vi "10.multi-dim-array.vi"() -> ()   [LabVIEW 2016]
panel:
  out "Array 3":dbl[][](array[numeric])
  out "Array 2":dbl[][](array[numeric])
  in  "Array1":dbl[][](array[numeric])
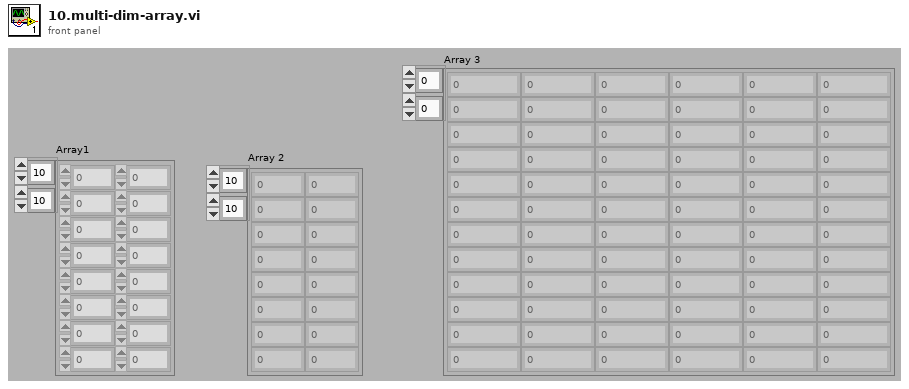
[diagram p1: front panel]
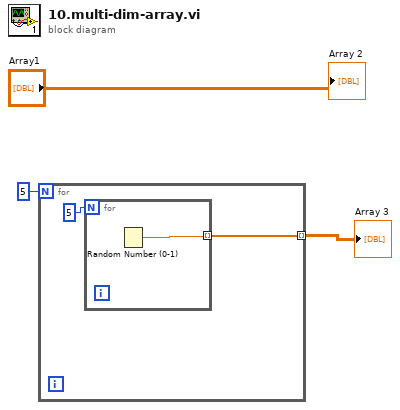
[diagram p0: block diagram]
diagram:
  n1 = for {
    N: 5 -> [_]
    tunnel: [w5] -> w1 mode=indexing
    n2 = for {
      N: 5 -> [_]
      tunnel: [w6] -> w5 mode=indexing
      n3 = Random Number (0-1)() -> (number: 0 to 1=w6:dbl)
    }
  }
  "Array 3" <- w1
  "Array 2" <- "Array1"
